vi "is ROI Empty.vi"(2 "Current ROI Descriptor":T1 {"Contours"."Type" items=["No Selection", "Point", "Line", "Rectangle", "Oval", "Polygon", "Freehand Region", "Annulus", "Unused2", "Unused3", "Broken Line", "Freehand Line", "Rotated Rectangle"]}) -> (7 "Empty ROI?":bool)   [LabVIEW 2021, in "Image.lvlib"]
uses:
  Image.lvlib
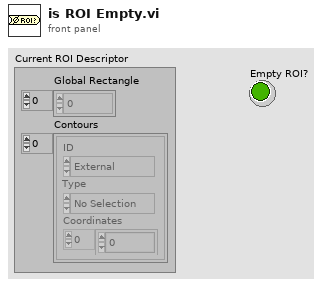
[diagram p1: front panel]
types:
  T1 = typedef "ROI Descriptor" = cluster{"Global Rectangle":i32[], "Contours":cluster{"ID":enum32{"External", "Internal"}, "Type":u32, "Coordinates":i32[]}[]}
  T2 = cluster{"ID":enum32{"External", "Internal"}, "Type":u32, "Coordinates":i32[]}[]
  T3 = cluster{"ID":enum32{"External", "Internal"}, "Type":u32, "Coordinates":i32[]}
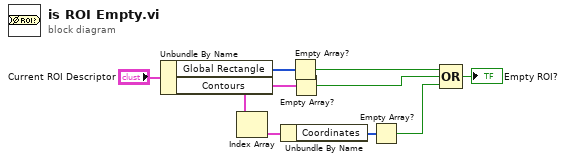
[diagram p0: block diagram]
diagram:
  n1 = Unbundle By Name("Current ROI Descriptor") -> ("Global Rectangle"=w8:i32[], "Contours"=w7:T2)
  n2 = Index Array(array=w7) -> (element=w6:T3)  [unwired: 1 in]
  n3 = Unbundle By Name(w6) -> ("Coordinates"=w5:i32[])
  n4 = Empty Array?(array=w8) -> (empty?=w4:bool)
  n5 = Empty Array?(array=w7) -> (empty?=w3:bool)
  n6 = Empty Array?(array=w5) -> (empty?=w2:bool)
  n7 = Compound Arithmetic op=OR(w4, w3, w2) -> (→"Empty ROI?":bool)
